vi "create_RunSripts_menu.vi"(11 "menu reference":refnum<k9>) -> ()   [LabVIEW 2015]
doc: "Gets the names of all the script files inside the RunScripts Folder and creates the RunScripts Menu entries"
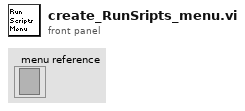
[diagram p1: front panel]
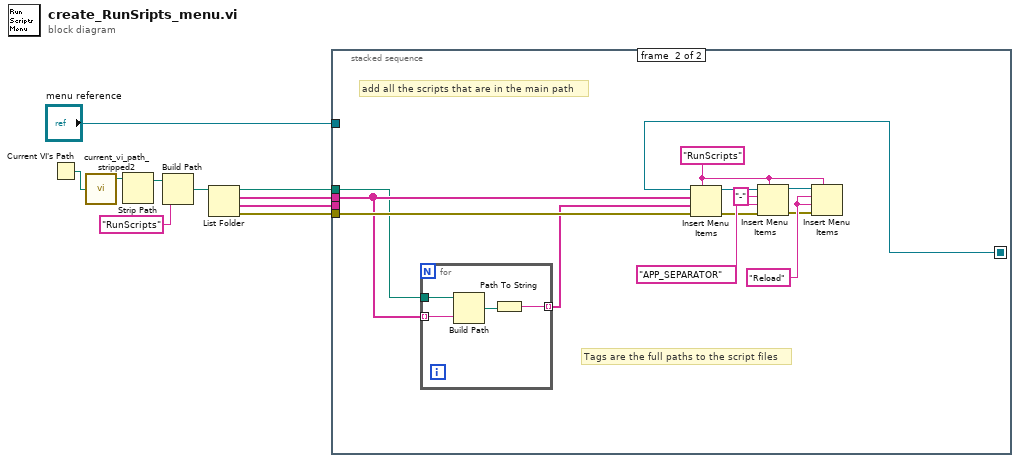
[diagram p0: block diagram]
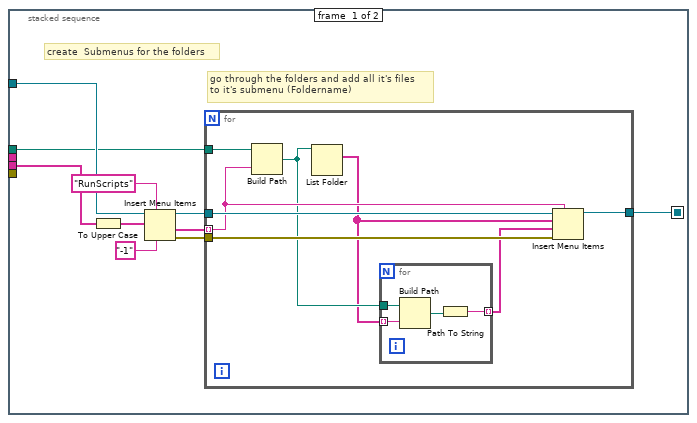
[diagram p2: hidden frame]
diagram:
  n1 = Current VI's Path() -> (path=w6:path)
  n2 = call "current_vi_path_stripped2.vi"("current VI Path"=w6) -> ("current VI Path stripped out"=w10:path)  [unwired: 3 in, 1 out]
  n3 = Strip Path(path=w10) -> (stripped path=w9:path)  [unwired: 1 out]
  n4 = Build Path(base path=w9, name or relative path="RunScripts") -> (appended path=w8:path)
  n5 = List Folder(path=w8) -> (path out=w2:path, filenames=w5:string[], folder names=w3:string[], error out=w4:errorcluster)  [unwired: 3 in]
  n6 = stacked-sequence {
    seq-local: [w13 _] -> [_ w36]
    tunnel: w5 -> [_ w35]
    tunnel: w4 -> [_ w37]
    tunnel: "menu reference" -> [w20 _]
    tunnel: w3 -> [w15 _]
    tunnel: w2 -> [w16 w34]
    frame #0 {
      # "go through the folders and add all it's files\nto it's submenu (Foldername)"
      # "create  Submenus for the folders"
      n7 = To Upper Case(1:w15) -> (0:w14:string[])
      n8 = Insert Menu Items(4:"-1" ("after item"), 5:"RunScripts" ("menu tag"), 8:w14, 9:w20) -> (0:w18:errorcluster, 1:w17:string[], 3:w19:refnum<k9>)  [unwired: 2 in]
      n9 = for {
        tunnel: w19 -> [w27]
        tunnel: w18 -> [w26]
        tunnel: w17 -> [w25] mode=indexing
        tunnel: w16 -> [w28]
        tunnel: [w24] -> w13
        n10 = Build Path(base path=w28, name or relative path=w25) -> (appended path=w23:path)
        n11 = List Folder(path=w23) -> (filenames=w22:string[])  [unwired: 3 in, 3 out]
        n12 = for {
          tunnel: w23 -> [w32]
          tunnel: w22 -> [w31] mode=indexing
          tunnel: [w29] -> w21 mode=indexing
          n13 = Build Path(base path=w32, name or relative path=w31) -> (appended path=w30:path)
          n14 = Path To String(path=w30) -> (string=w29:string)
        }
        n15 = Insert Menu Items(5:w25, 6:w26, 7:w21, 8:w22, 9:w27) -> (3:w24:refnum<k9>)  [unwired: 1 in, 2 out]
      }
    }
    frame #1 {
      w45 = "Reload" ("menu tag")
      w44 = "RunScripts" ("menu tag")
      # "Tags are the full paths to the script files"
      # "add all the scripts that are in the main path"
      n16 = for {
        tunnel: w35 -> [w47] mode=indexing
        tunnel: w34 -> [w48]
        tunnel: [w46] -> w33 mode=indexing
        n17 = Build Path(base path=w48, name or relative path=w47) -> (appended path=w49:path)
        n18 = Path To String(path=w49) -> (string=w46:string)
      }
      n19 = Insert Menu Items(5:w44, 6:w37, 7:w33, 8:w35, 9:w36) -> (0:w38:errorcluster, 3:w39:refnum<k9>)  [unwired: 1 in, 1 out]
      n20 = Insert Menu Items(5:w44, 6:w38, 7:"APP_SEPARATOR" ("menu tag"), 8:"-" ("item names"), 9:w39) -> (0:w42:errorcluster, 3:w43:refnum<k9>)  [unwired: 1 in, 1 out]
      n21 = Insert Menu Items(5:w44, 6:w42, 7:w45, 8:w45, 9:w43) -> ()  [unwired: 1 in, 3 out]
    }
  }
